vi "Stop Core.vi"(10 "final error code":i32, 11 "Calibration Actor in":refnum<class "Calibration Actor.lvclass">) -> (3 "Calibration Actor out":refnum<class "Calibration Actor.lvclass">)   [LabVIEW 2014, in "Calibration.lvlib" / "Calibration Actor.lvclass"]
doc: "(<B>Filename</B>: Actor Framework.lvlib:Actor.lvclass:Stop Core.vi)\n\nDefines what the actor does before it stops. Use the <B>final error code</B> input to determine whether the actor shut down in response to an error.\n\nBy default, this method does nothing. A descendant class may override it to define behavior, such as shutting down any processes the actor initiated in its override of the Actor Core method."
uses:
  Calibration Actor.lvclass
  <vilib>/ActorFramework/Actor/Actor.lvclass/Actor.ctl
  Calibration Actor.lvclass/Calibration Actor.ctl
  Controller/Messages/Toggle Filter Cycle/Toggle Filter Cycle MSG.lvclass
  Controller/Messages/Toggle Speaker Cycle/Toggle Speaker Cycle MSG.lvclass
  Controller/Messages/Update Device Setpoint MSG/Update Device Setpoint.lvclass
  Controller/Messages/O3 Valve MSG/O3 Valve MSG.lvclass
  Controller/Messages/Change Filter State/Change Filter State.lvclass
  Controller/Messages/Change Speaker MSG/Speaker MSG.lvclass
  Controller/Messages/Update Switch State MSG/Update Switch MSG.lvclass/Update Switch MSG.ctl
  Controller/Messages/Change Speaker MSG/Speaker MSG.lvclass/Speaker MSG.ctl
  Controller/Messages/Toggle Speaker Cycle/Toggle Speaker Cycle MSG.lvclass/Toggle Speaker Cycle MSG.ctl
  Controller/Messages/Toggle Filter Cycle/Toggle Filter Cycle MSG.lvclass/Toggle Filter Cycle MSG.ctl
  Controller/Messages/Update Device Setpoint MSG/Update Device Setpoint.lvclass/Update Device Setpoint.ctl
  SuperActor/SuperActor.lvclass/SuperActor.ctl
  <vilib>/ActorFramework/Message Enqueuer/Message Enqueuer.lvclass/Message Enqueuer.ctl
  Read Cal Type.vi
  SuperActor/Read Log Session.vi
  SuperActor/Read CVT Session.vi
  Controller/Messages/Update Switch State MSG/Write SwitchState.vi
  Controller/Messages/Change Speaker MSG/Write spk.vi
  Controller/Messages/Toggle Speaker Cycle/Write Cycle_.vi
  Controller/Messages/Toggle Filter Cycle/Write Cycle_.vi
  Controller/Messages/Update Device Setpoint MSG/Write DevID.vi
  Controller/Messages/Update Device Setpoint MSG/Write SP.vi
  <vilib>/ActorFramework/Message Priority Queue/Priority Enqueue.vi
  SuperActor/SuperActor.lvclass
  <userlib>/_Session Fwk/Session - Root.lvclass
  reusable/Session APIs/Session Log/System Log.lvclass
  <vilib>/ActorFramework/Actor/Actor.lvclass
  <vilib>/ActorFramework/Message Enqueuer/Message Enqueuer.lvclass
  reusable/Session APIs/CVT/CVT.lvclass
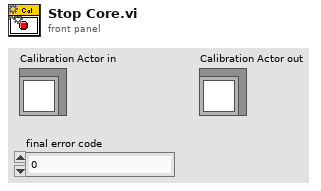
[diagram p1: front panel]
types:
  T1 = typedef "Session - Root.lvclass/Session Handle.ctl" = refnum<data-value>
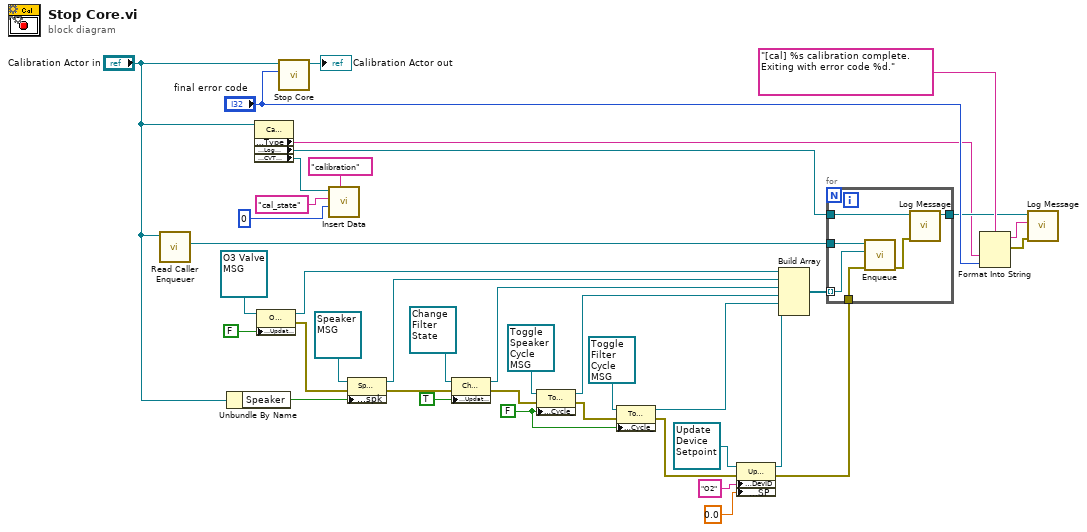
[diagram p0: block diagram]
diagram:
  w26 = FALSE ("Cycle_")
  n1 = call <vilib>:"Read Caller Enqueuer.vi"("Actor"="Calibration Actor in") -> ("Caller Enqueuer"=w25:refnum<class "Message Enqueuer.lvclass">)  [unwired: 10 in]
  n2 = Unbundle By Name("Calibration Actor in") -> ("Speaker"=w30:bool)
  n3 = property class="Calibration Actor"(reference="Calibration Actor in") -> ("Accessors:Type"=w1:string, "Accessors:Log Session"=w2:T1, "Accessors:CVT Session"=w7:T1)  [unwired: 1 in, 2 out]
  n4 = property class="O3 Valve"(reference=refnum<class "O3 Valve MSG.lvclass"> refnum ("Controller:O3 Valve"), "Accessors:UpdateSw"=FALSE ("Val")) -> (reference out=w23:refnum<class "O3 Valve MSG.lvclass">, error out=w13:errorcluster)  [unwired: 1 in]
  n5 = call-parent "Stop Core.vi"("final error code"="final error code", "Ex Nested in"="Calibration Actor in") -> ("Ex Nested out"=→"Calibration Actor out":refnum<class "Calibration Actor.lvclass">)  [unwired: 9 in]
  n6 = call "Insert Data.vi"("Group"="calibration", "Data"=u8 0, "tag"="cal_state", "CVT Session In"=w7) -> ()  [unwired: 6 in, 2 out]
  n7 = property class="Speaker MSG.lvclass"(reference=refnum<class "Speaker MSG.lvclass"> refnum ("Controller:Speaker MSG.lvclass"), error in=w13, "Accessors:spk"=w30) -> (reference out=w22:refnum<class "Speaker MSG.lvclass">, error out=w12:errorcluster)
  n8 = property class="Change Filter State MSG"(reference=refnum<class "Change Filter State.lvclass"> refnum ("Controller:Change Filter State MSG"), error in=w12, "Accessors:UpdateSw"=TRUE ("UpdateSw")) -> (reference out=w21:refnum<class "Change Filter State.lvclass">, error out=w11:errorcluster)
  n9 = property class="Toggle Speaker Cycle MSG"(reference=refnum<class "Toggle Speaker Cycle MSG.lvclass"> refnum ("Controller:Toggle Speaker Cycle MSG"), error in=w11, "Accessors:Cycle_"=w26) -> (reference out=w20:refnum<class "Toggle Speaker Cycle MSG.lvclass">, error out=w10:errorcluster)
  n10 = property class="Toggle Filter Cycle"(reference=refnum<class "Toggle Filter Cycle MSG.lvclass"> refnum ("Controller:Toggle Filter Cycle MSG.lvclass"), error in=w10, "Accessors:Cycle_"=w26) -> (reference out=w19:refnum<class "Toggle Filter Cycle MSG.lvclass">, error out=w9:errorcluster)
  n11 = property class="Update Device Setpoint"(reference=refnum<class "Update Device Setpoint.lvclass"> refnum ("Controller:Update Device Setpoint"), error in=w9, "Accessors:DevID"="O2" ("DevID"), "Accessors:SP"=0.0 ("SP")) -> (reference out=w15:refnum<class "Update Device Setpoint.lvclass">, error out=w8:errorcluster)
  n12 = Build Array(w23, w22, w21, w20, w19, w15) -> (w14:refnum<class "Message.lvclass">[])
  n13 = for {
    tunnel: w25 -> [w45]
    tunnel: w2 -> [w44]
    tunnel: [w43] -> w24
    tunnel: w14 -> [w41] mode=indexing
    tunnel: w8 -> [w40]
    n14 = call <vilib>:"Enqueue.vi"("error in (no error)"=w40, "Message"=w41, "Message Enqueuer in"=w45) -> ("error out"=w42:errorcluster)  [unwired: 7 in, 1 out]
    n15 = call "Log Message.vi"("error in"=w42, "session in"=w44) -> ("session out"=w43:T1)  [unwired: 8 in, 1 out]
  }
  n16 = Format Into String(format string="[cal] %s calibration complete.  Exiting with error code %d.", w1, "final error code") -> (resulting string=w37:string, error out=w36:errorcluster)  [unwired: 2 in]
  n17 = call "Log Message.vi"("error in"=w36, "MSG In"=w37, "session in"=w24) -> ()  [unwired: 7 in, 2 out]
